vi "map_XY_frame.vi"() -> ()   [LabVIEW 2015]
panel:
  in  "move z":bool
  in  "Z step":string
  in  "goto y pos 2":bool
  in  "y move 2":string
  in  "goto x pos 2":bool
  in  "X move 2":string
  in  "t speed":string="10"
  in  "t step":string="3"
  in  "y speed":string="20"
  in  "y step":string
  in  "x speed":string="20"
  in  "x step":string="100"
  in  "start":bool
  in  "n frame":string
  in  "passo frame":string
  in  "length":string
  out "String":string
  in  "KILL":bool
  in  "PAUSE":bool
  in  "RESUME":bool
  in  "QUIT":bool
  in  "Done":bool
  in  "End":bool
  in  "zero z - end":bool
  in  "zero x - end":bool
  in  "zero y - end":bool
  out "output":string
  out "command":string
  in  "zero done":bool
  in  "zero z":bool
  in  "zero x":bool
  in  "zero y":bool
  # "Comandi di emergenza"
  # "MAPPING XY STIFFBACK"
  # "Posiziono in zero"
  # "Vado sulla piastra \ne azzero"
  # "Ritorno a zero"
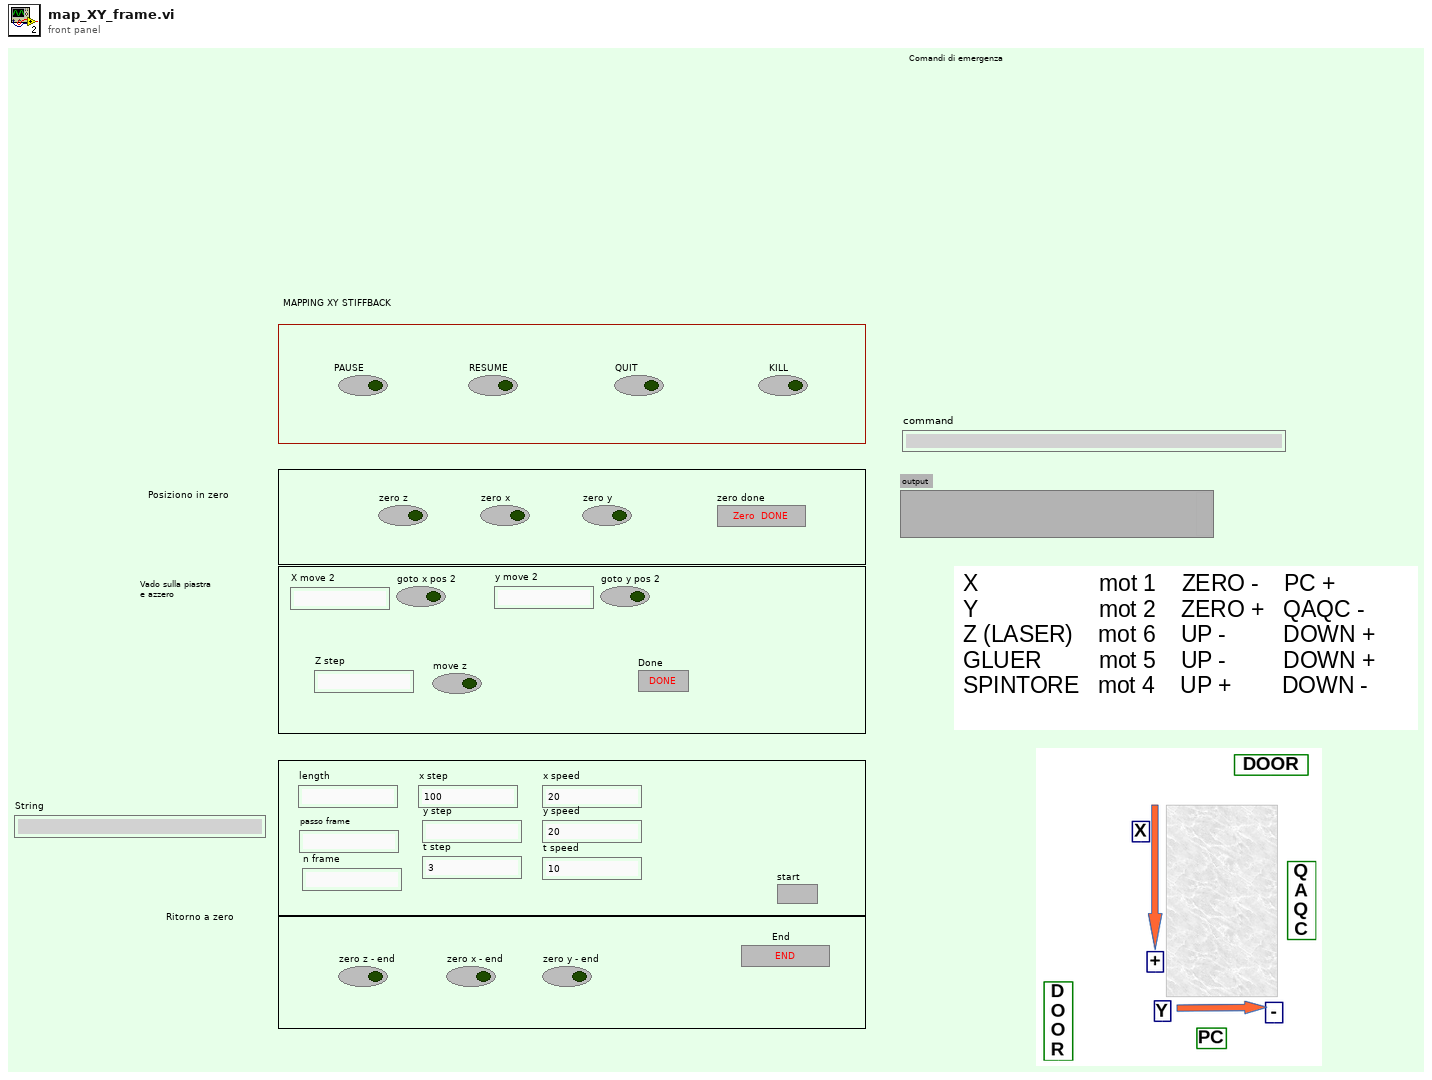
[diagram p1: front panel]
types:
  T1 = enum16{"open", "replace", "create", "open or create", "replace or create", "replace or create with confirmation"}
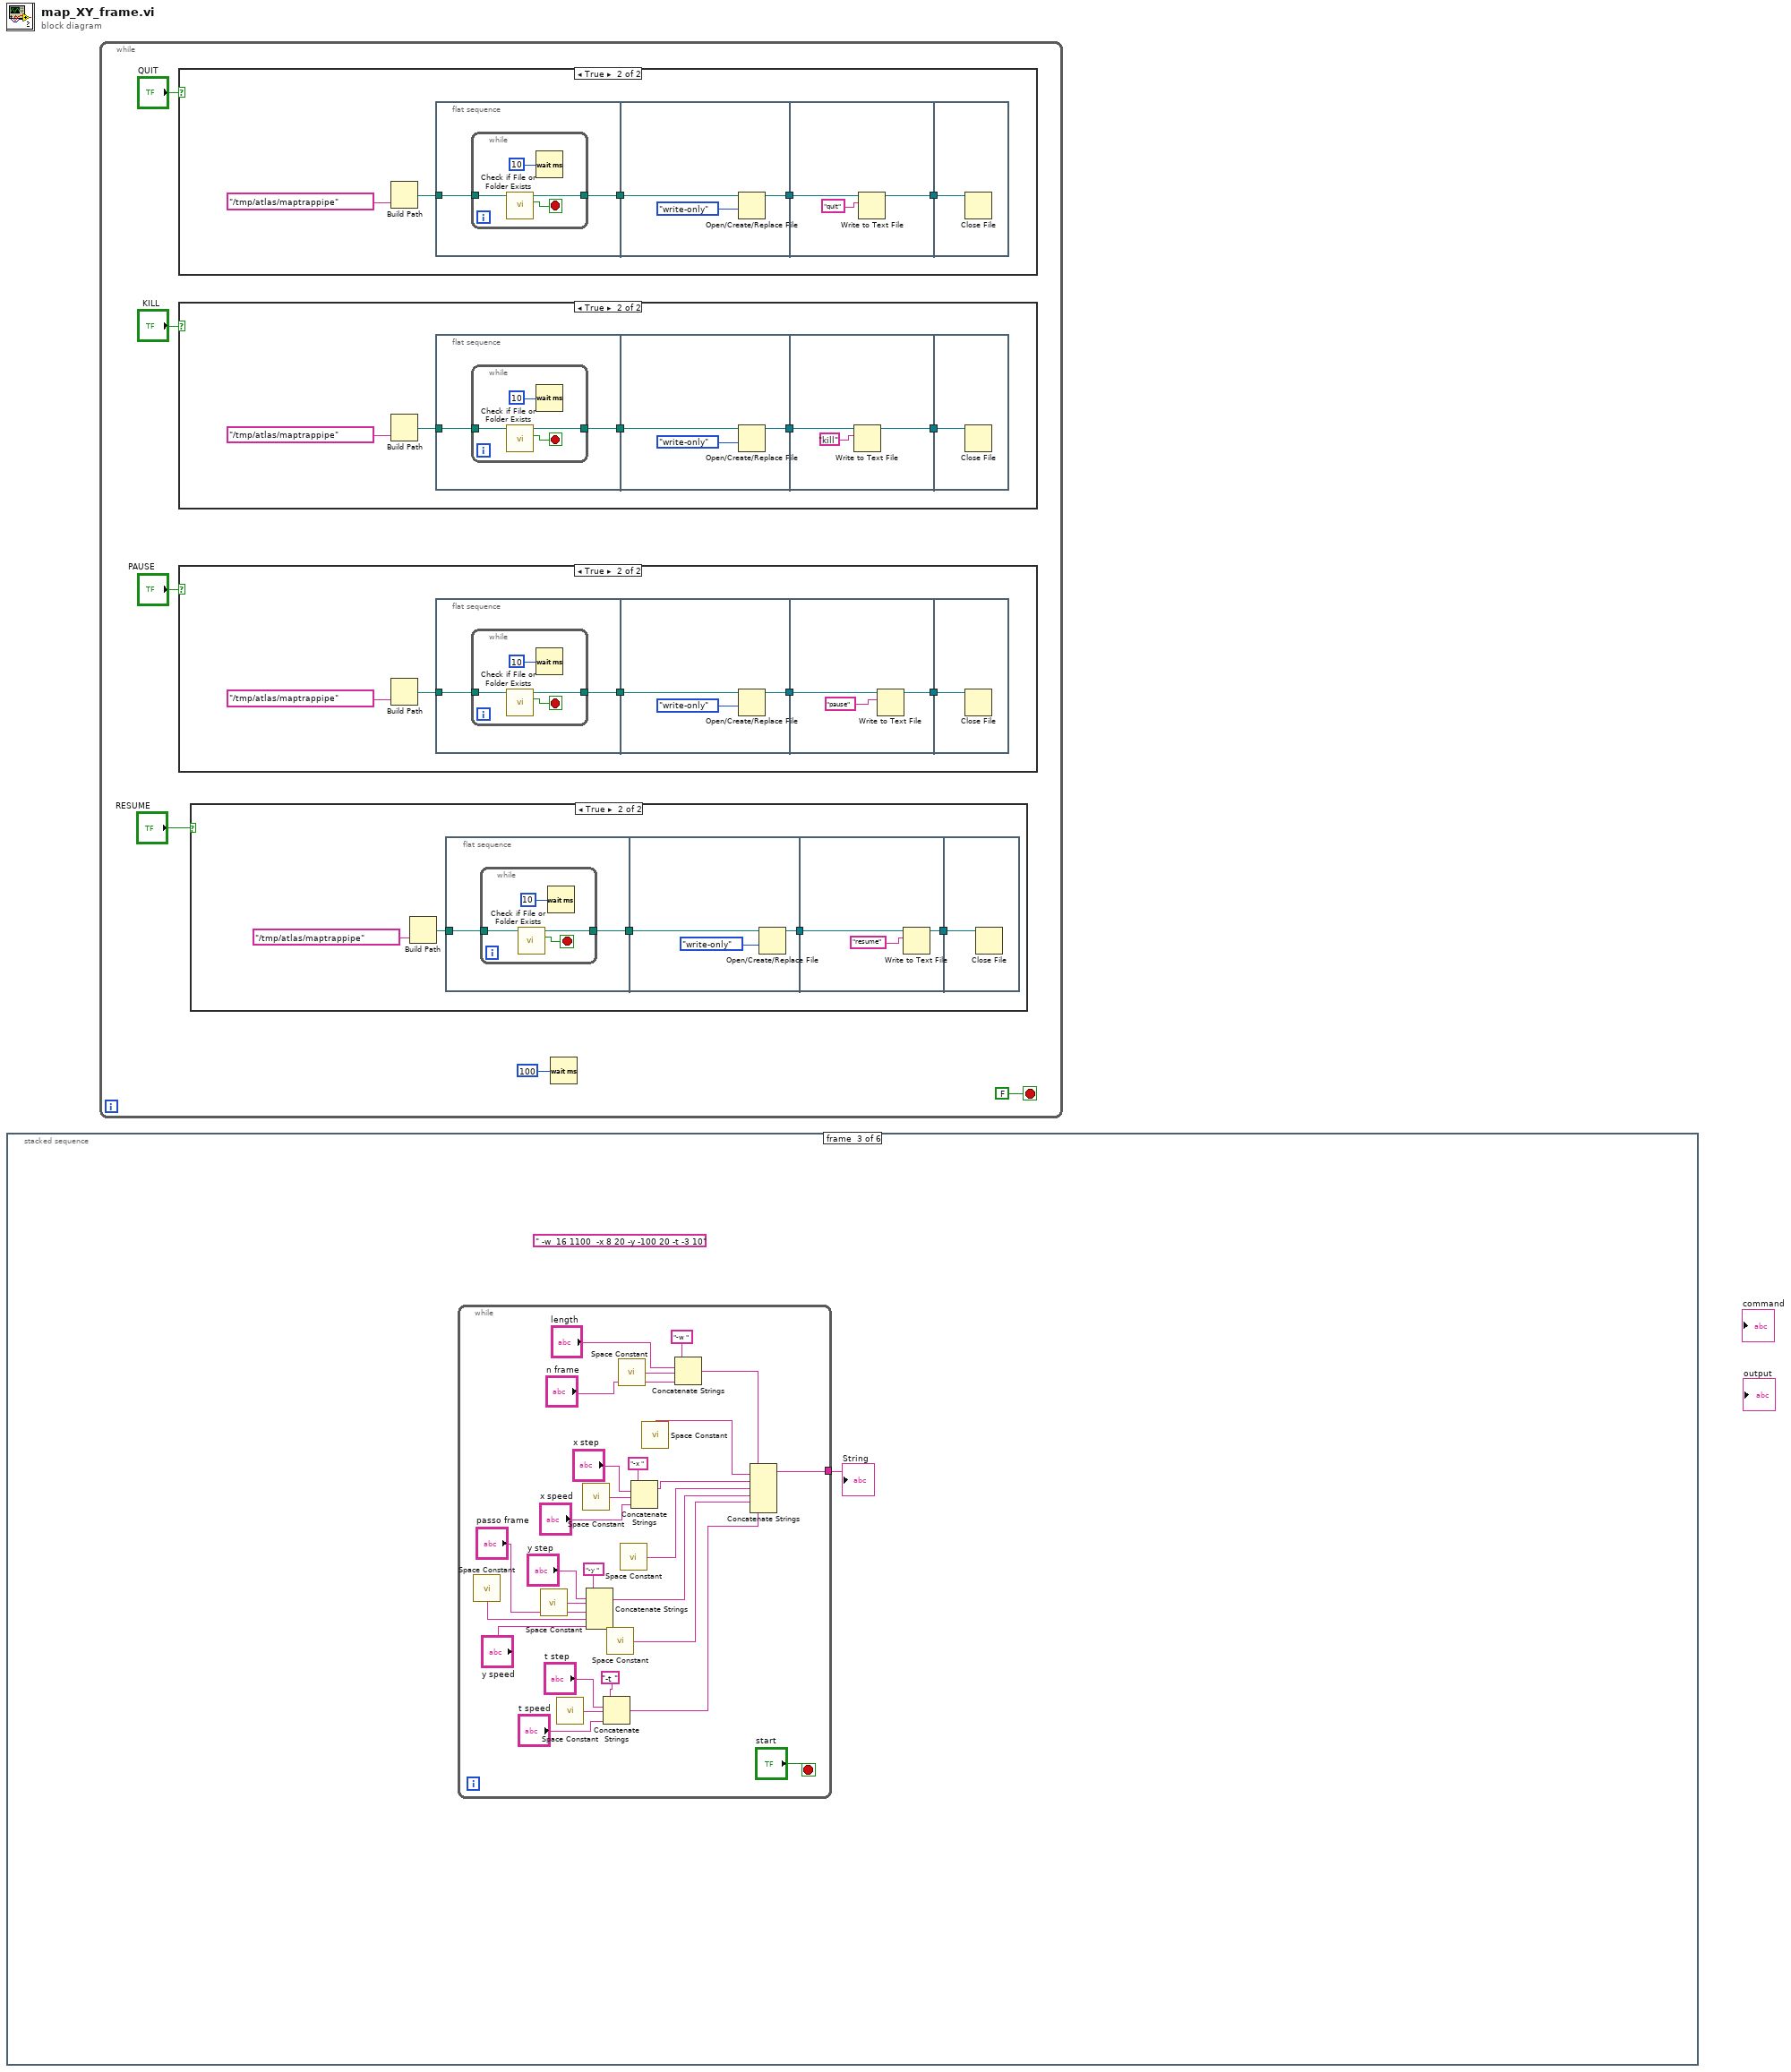
[diagram p0: block diagram]
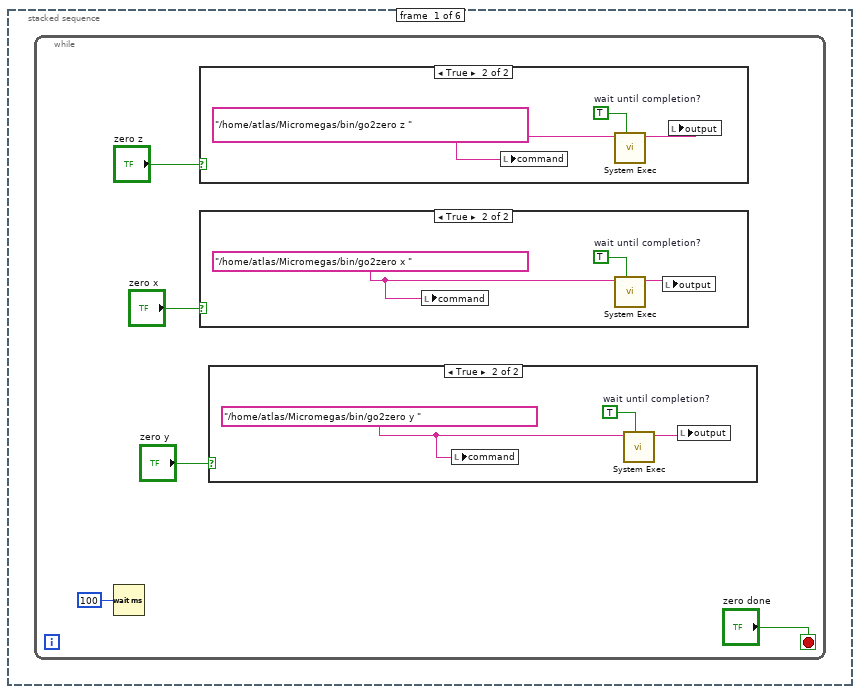
[diagram p6: hidden frame]
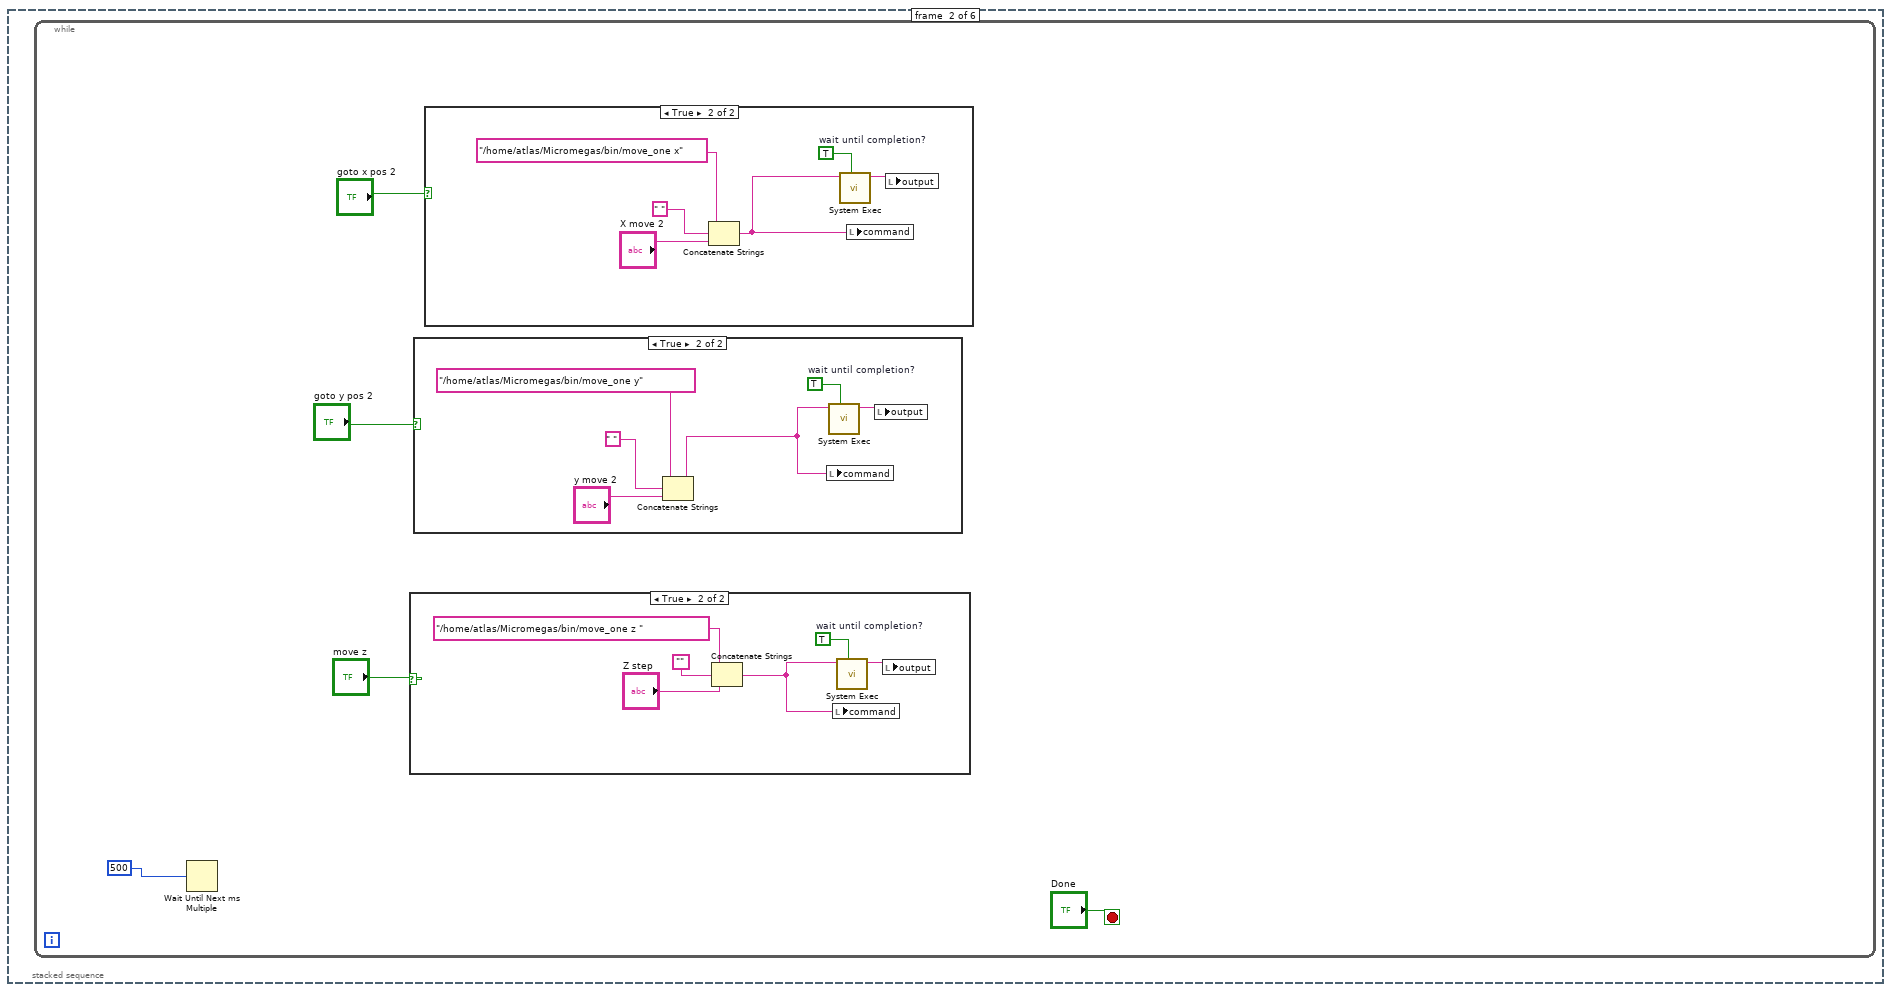
[diagram p10: hidden frame]
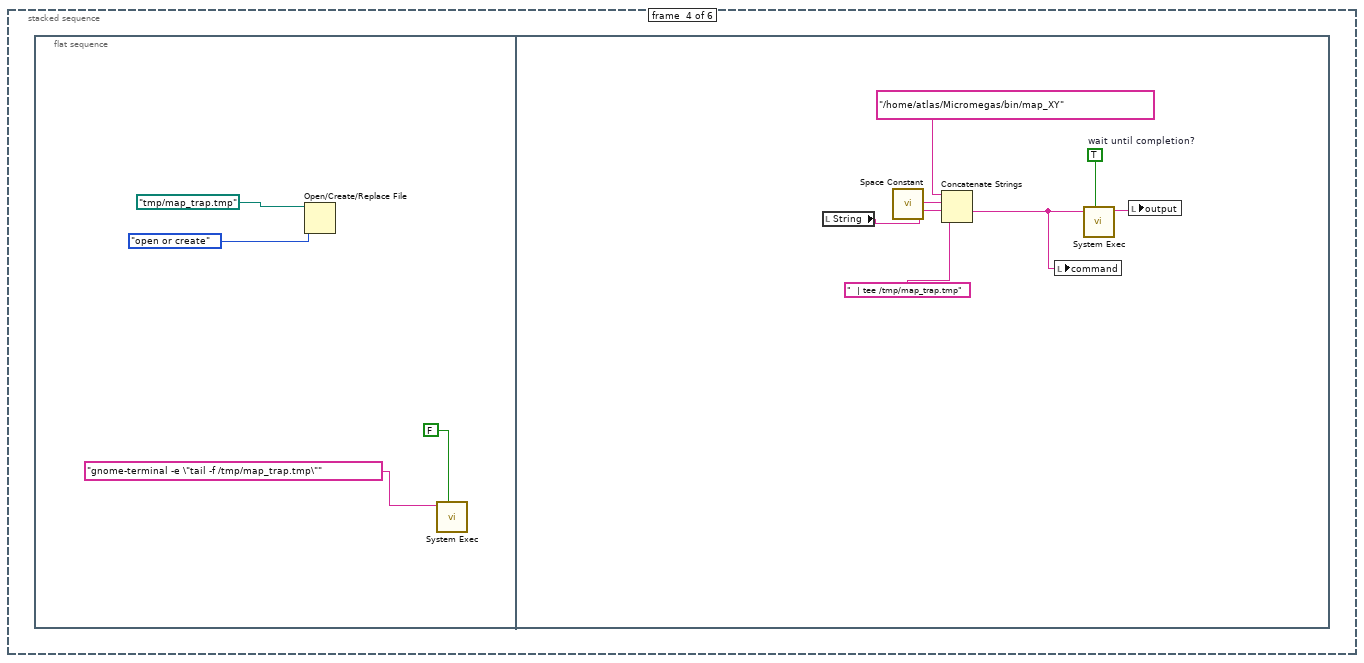
[diagram p14: hidden frame]
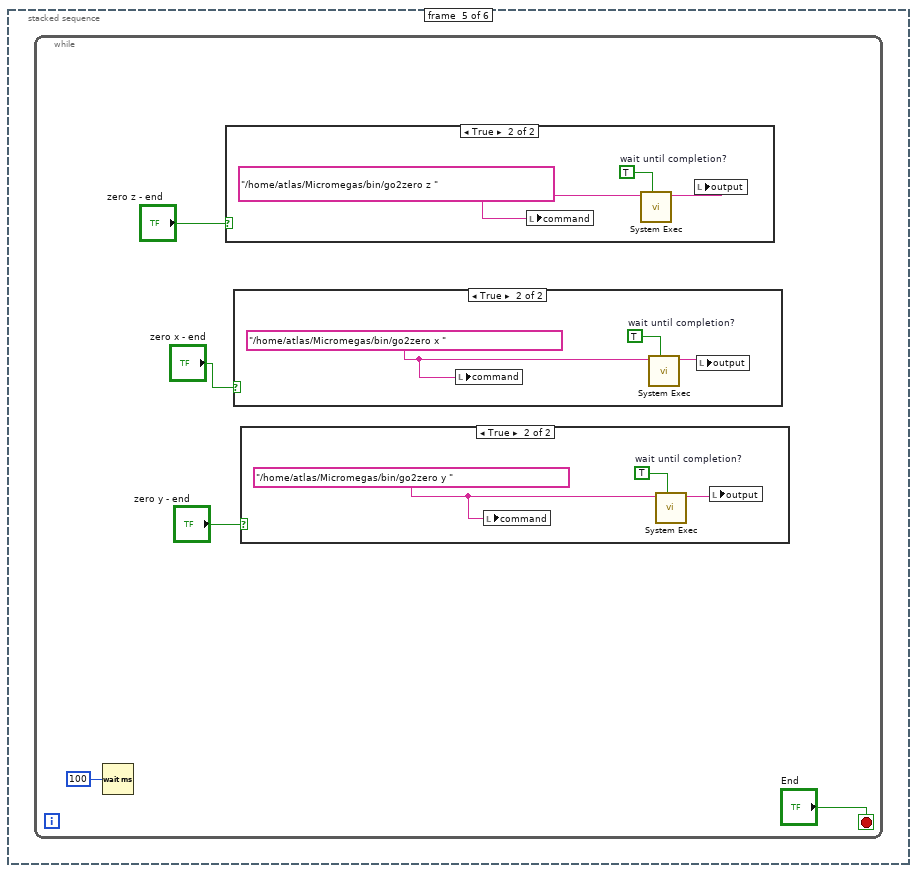
[diagram p15: hidden frame]
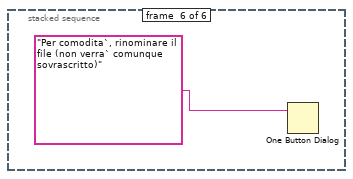
[diagram p19: hidden frame]
diagram:
  n1 = stacked-sequence {
    frame #0 {
      n2 = while {
        stop <- "zero done" stop-if-true
        n3 = Wait (ms)(milliseconds to wait=u32 100) -> ()  [unwired: 1 out]
        n4 = case shown="True" "zero z" {
          frame False {
          }
          frame True {
            w13 = "/home/atlas/Micromegas/bin/go2zero z " ("string")
            w14 = TRUE  # wait until completion?
            n5 = local write "command"(w13) -> ()
            n6 = call <vilib>:"System Exec.vi"("wait until completion? (T)"=w14, "command line"=w13) -> ("standard output"=w12:string)  [unwired: 6 in, 3 out]
            n7 = local write "output"(w12) -> ()
          }
        }
        n8 = case shown="True" "zero x" {
          frame False {
          }
          frame True {
            w10 = "/home/atlas/Micromegas/bin/go2zero x " ("string")
            w11 = TRUE  # wait until completion?
            n9 = local write "command"(w10) -> ()
            n10 = call <vilib>:"System Exec.vi"("wait until completion? (T)"=w11, "command line"=w10) -> ("standard output"=w9:string)  [unwired: 6 in, 3 out]
            n11 = local write "output"(w9) -> ()
          }
        }
        n12 = case shown="True" "zero y" {
          frame False {
          }
          frame True {
            w7 = "/home/atlas/Micromegas/bin/go2zero y " ("string")
            w8 = TRUE  # wait until completion?
            n13 = local write "command"(w7) -> ()
            n14 = call <vilib>:"System Exec.vi"("wait until completion? (T)"=w8, "command line"=w7) -> ("standard output"=w6:string)  [unwired: 6 in, 3 out]
            n15 = local write "output"(w6) -> ()
          }
        }
      }
    }
    frame #1 {
      n16 = while {
        stop <- "Done" stop-if-true
        n17 = Wait Until Next ms Multiple(millisecond multiple=u32 500 ("millisecond timer value")) -> ()  [unwired: 1 out]
        n18 = case shown="True" "move z" {
          frame False {
          }
          frame True {
            w25 = TRUE  # wait until completion?
            n19 = Concatenate Strings("/home/atlas/Micromegas/bin/move_one z " ("string"), "", "Z step") -> (w20:string)
            n20 = local write "command"(w20) -> ()
            n21 = call <vilib>:"System Exec.vi"("wait until completion? (T)"=w25, "command line"=w20) -> ("standard output"=w24:string)  [unwired: 6 in, 3 out]
            n22 = local write "output"(w24) -> ()
          }
        }
        n23 = case shown="True" "goto y pos 2" {
          frame False {
          }
          frame True {
            w31 = TRUE  # wait until completion?
            n24 = Concatenate Strings("/home/atlas/Micromegas/bin/move_one y" ("string"), " ", "y move 2") -> (w27:string)
            n25 = local write "command"(w27) -> ()
            n26 = call <vilib>:"System Exec.vi"("wait until completion? (T)"=w31, "command line"=w27) -> ("standard output"=w30:string)  [unwired: 6 in, 3 out]
            n27 = local write "output"(w30) -> ()
          }
        }
        n28 = case shown="True" "goto x pos 2" {
          frame False {
          }
          frame True {
            w37 = TRUE  # wait until completion?
            n29 = Concatenate Strings("/home/atlas/Micromegas/bin/move_one x" ("string"), " ", "X move 2") -> (w33:string)
            n30 = call <vilib>:"System Exec.vi"("wait until completion? (T)"=w37, "command line"=w33) -> ("standard output"=w36:string)  [unwired: 6 in, 3 out]
            n31 = local write "command"(w33) -> ()
            n32 = local write "output"(w36) -> ()
          }
        }
      }
    }
    frame #2 {
      (unwired) " -w  16 1100  -x 8 20 -y -100 20 -t -3 10" ("string")
      n33 = while {
        tunnel: [w49] -> w38
        stop <- "start" stop-if-true
        n34 = call <vilib>:"Space Constant.vi"() -> ("String"=w39:string)
        n35 = call <vilib>:"Space Constant.vi"() -> ("String"=w54:string)
        n36 = call <vilib>:"Space Constant.vi"() -> ("String"=w51:string)
        n37 = call <vilib>:"Space Constant.vi"() -> ("String"=w58:string)
        n38 = Concatenate Strings("-y ", "y step", w54, "passo frame", w39, "y speed") -> (w44:string)
        n39 = Concatenate Strings("-t ", "t step", w51, "t speed") -> (w42:string)
        n40 = call <vilib>:"Space Constant.vi"() -> ("String"=w43:string)
        n41 = call <vilib>:"Space Constant.vi"() -> ("String"=w63:string)
        n42 = call <vilib>:"Space Constant.vi"() -> ("String"=w45:string)
        n43 = Concatenate Strings("-x ", "x step", w58, "x speed") -> (w46:string)
        n44 = call <vilib>:"Space Constant.vi"() -> ("String"=w47:string)
        n45 = Concatenate Strings("-w ", "length", w63, "n frame") -> (w48:string)
        n46 = Concatenate Strings(w48, w47, w46, w45, w44, w43, w42) -> (w49:string)
      }
      "String" <- w38
    }
    frame #3 {
      n47 = flat-sequence {
        frame #0 {
          n48 = Open/Create/Replace File(file path (use dialog)=path "/tmp/map_trap.tmp", operation (0:open)=T1."open or create") -> ()  [unwired: 4 in, 3 out]
          n49 = call <vilib>:"System Exec.vi"("wait until completion? (T)"=FALSE, "command line"="gnome-terminal -e \"tail -f /tmp/map_trap.tmp\"") -> ()  [unwired: 6 in, 4 out]
        }
        frame #1 {
          w76 = TRUE  # wait until completion?
          n50 = local read "String"() -> (w70:string)
          n51 = call <vilib>:"Space Constant.vi"() -> ("String"=w74:string)
          n52 = Concatenate Strings("/home/atlas/Micromegas/bin/map_XY" ("string"), w74, w70, "  | tee /tmp/map_trap.tmp" ("string")) -> (w72:string)
          n53 = local write "command"(w72) -> ()
          n54 = call <vilib>:"System Exec.vi"("wait until completion? (T)"=w76, "command line"=w72) -> ("standard output"=w71:string)  [unwired: 6 in, 3 out]
          n55 = local write "output"(w71) -> ()
        }
      }
    }
    frame #4 {
      n56 = while {
        stop <- "End" stop-if-true
        n57 = Wait (ms)(milliseconds to wait=u32 100) -> ()  [unwired: 1 out]
        n58 = case shown="True" "zero z - end" {
          frame False {
          }
          frame True {
            w89 = "/home/atlas/Micromegas/bin/go2zero z " ("string")
            w90 = TRUE  # wait until completion?
            n59 = local write "command"(w89) -> ()
            n60 = call <vilib>:"System Exec.vi"("wait until completion? (T)"=w90, "command line"=w89) -> ("standard output"=w88:string)  [unwired: 6 in, 3 out]
            n61 = local write "output"(w88) -> ()
          }
        }
        n62 = case shown="True" "zero x - end" {
          frame False {
          }
          frame True {
            w86 = "/home/atlas/Micromegas/bin/go2zero x " ("string")
            w87 = TRUE  # wait until completion?
            n63 = local write "command"(w86) -> ()
            n64 = call <vilib>:"System Exec.vi"("wait until completion? (T)"=w87, "command line"=w86) -> ("standard output"=w85:string)  [unwired: 6 in, 3 out]
            n65 = local write "output"(w85) -> ()
          }
        }
        n66 = case shown="True" "zero y - end" {
          frame False {
          }
          frame True {
            w83 = "/home/atlas/Micromegas/bin/go2zero y " ("string")
            w84 = TRUE  # wait until completion?
            n67 = local write "command"(w83) -> ()
            n68 = call <vilib>:"System Exec.vi"("wait until completion? (T)"=w84, "command line"=w83) -> ("standard output"=w82:string)  [unwired: 6 in, 3 out]
            n69 = local write "output"(w82) -> ()
          }
        }
      }
    }
    frame #5 {
      n70 = One Button Dialog(message="Per comodita`, rinominare il file (non verra` comunque sovrascritto)") -> ()  [unwired: 1 in, 1 out]
    }
  }
  n71 = while {
    stop <- FALSE stop-if-true
    n72 = case shown="True" "QUIT" {
      frame False {
      }
      frame True {
        n73 = Build Path(name or relative path="/tmp/atlas/maptrappipe" ("string")) -> (appended path=w152:path)  [unwired: 1 in]
        n74 = flat-sequence {
          tunnel: [w158] -> w156
          tunnel: w152 -> [w157]
          tunnel: w156 -> [w165]
          tunnel: [w163] -> w155
          tunnel: w155 -> [w168]
          tunnel: [w167] -> w154
          tunnel: w154 -> [w169]
          frame #0 {
            n75 = while {
              tunnel: [w160] -> w158
              tunnel: w157 -> [w159]
              stop <- w161 stop-if-true
              n76 = call <vilib>:"Check if File or Folder Exists.vi"("path"=w159) -> ("file or folder exists?"=w161:bool, "dup path"=w160:path)  [unwired: 8 in, 1 out]
              n77 = Wait (ms)(milliseconds to wait=u32 10) -> ()  [unwired: 1 out]
            }
          }
          frame #1 {
            n78 = Open/Create/Replace File(file path (use dialog)=w165, access (0:read/write)=enum16{"read/write", "read-only", "write-only"}."write-only") -> (refnum out=w163:refnum<file>)  [unwired: 4 in, 2 out]
          }
          frame #2 {
            n79 = Write to Text File(file (use dialog)=w168, text="quit") -> (refnum out=w167:refnum<file>)  [unwired: 2 in, 2 out]
          }
          frame #3 {
            n80 = Close File(refnum=w169) -> ()  [unwired: 1 in, 2 out]
          }
        }
      }
    }
    n81 = case shown="True" "KILL" {
      frame False {
      }
      frame True {
        n82 = Build Path(name or relative path="/tmp/atlas/maptrappipe" ("string")) -> (appended path=w116:path)  [unwired: 1 in]
        n83 = flat-sequence {
          tunnel: [w122] -> w120
          tunnel: w116 -> [w121]
          tunnel: w120 -> [w129]
          tunnel: [w127] -> w119
          tunnel: w119 -> [w132]
          tunnel: [w131] -> w118
          tunnel: w118 -> [w133]
          frame #0 {
            n84 = while {
              tunnel: [w124] -> w122
              tunnel: w121 -> [w123]
              stop <- w125 stop-if-true
              n85 = call <vilib>:"Check if File or Folder Exists.vi"("path"=w123) -> ("file or folder exists?"=w125:bool, "dup path"=w124:path)  [unwired: 8 in, 1 out]
              n86 = Wait (ms)(milliseconds to wait=u32 10) -> ()  [unwired: 1 out]
            }
          }
          frame #1 {
            n87 = Open/Create/Replace File(file path (use dialog)=w129, access (0:read/write)=enum16{"read/write", "read-only", "write-only"}."write-only") -> (refnum out=w127:refnum<file>)  [unwired: 4 in, 2 out]
          }
          frame #2 {
            n88 = Write to Text File(file (use dialog)=w132, text="kill") -> (refnum out=w131:refnum<file>)  [unwired: 2 in, 2 out]
          }
          frame #3 {
            n89 = Close File(refnum=w133) -> ()  [unwired: 1 in, 2 out]
          }
        }
      }
    }
    n90 = case shown="True" "PAUSE" {
      frame False {
      }
      frame True {
        n91 = Build Path(name or relative path="/tmp/atlas/maptrappipe" ("string")) -> (appended path=w98:path)  [unwired: 1 in]
        n92 = flat-sequence {
          tunnel: [w104] -> w102
          tunnel: w98 -> [w103]
          tunnel: w102 -> [w111]
          tunnel: [w109] -> w101
          tunnel: w101 -> [w114]
          tunnel: [w113] -> w100
          tunnel: w100 -> [w115]
          frame #0 {
            n93 = while {
              tunnel: [w106] -> w104
              tunnel: w103 -> [w105]
              stop <- w107 stop-if-true
              n94 = call <vilib>:"Check if File or Folder Exists.vi"("path"=w105) -> ("file or folder exists?"=w107:bool, "dup path"=w106:path)  [unwired: 8 in, 1 out]
              n95 = Wait (ms)(milliseconds to wait=u32 10) -> ()  [unwired: 1 out]
            }
          }
          frame #1 {
            n96 = Open/Create/Replace File(file path (use dialog)=w111, access (0:read/write)=enum16{"read/write", "read-only", "write-only"}."write-only") -> (refnum out=w109:refnum<file>)  [unwired: 4 in, 2 out]
          }
          frame #2 {
            n97 = Write to Text File(file (use dialog)=w114, text="pause") -> (refnum out=w113:refnum<file>)  [unwired: 2 in, 2 out]
          }
          frame #3 {
            n98 = Close File(refnum=w115) -> ()  [unwired: 1 in, 2 out]
          }
        }
      }
    }
    n99 = case shown="True" "RESUME" {
      frame False {
      }
      frame True {
        n100 = Build Path(name or relative path="/tmp/atlas/maptrappipe" ("string")) -> (appended path=w134:path)  [unwired: 1 in]
        n101 = flat-sequence {
          tunnel: [w140] -> w138
          tunnel: w134 -> [w139]
          tunnel: w138 -> [w147]
          tunnel: [w145] -> w137
          tunnel: w137 -> [w150]
          tunnel: [w149] -> w136
          tunnel: w136 -> [w151]
          frame #0 {
            n102 = while {
              tunnel: [w142] -> w140
              tunnel: w139 -> [w141]
              stop <- w143 stop-if-true
              n103 = call <vilib>:"Check if File or Folder Exists.vi"("path"=w141) -> ("file or folder exists?"=w143:bool, "dup path"=w142:path)  [unwired: 8 in, 1 out]
              n104 = Wait (ms)(milliseconds to wait=u32 10) -> ()  [unwired: 1 out]
            }
          }
          frame #1 {
            n105 = Open/Create/Replace File(file path (use dialog)=w147, access (0:read/write)=enum16{"read/write", "read-only", "write-only"}."write-only") -> (refnum out=w145:refnum<file>)  [unwired: 4 in, 2 out]
          }
          frame #2 {
            n106 = Write to Text File(file (use dialog)=w150, text="resume") -> (refnum out=w149:refnum<file>)  [unwired: 2 in, 2 out]
          }
          frame #3 {
            n107 = Close File(refnum=w151) -> ()  [unwired: 1 in, 2 out]
          }
        }
      }
    }
    n108 = Wait (ms)(milliseconds to wait=100) -> ()  [unwired: 1 out]
  }
